vi "Triggers-Stop.vi"(7 "Logging queue element":T1={"Imaging Protocol"=enum."Live Imaging", "Number of Trials"=0, "Frame Size"=512, "# Averaged frames"=0, "Dwell time (us)"=0.0, "Index of Z-plane"=0, "Timelapse?"=FALSE, "Logging process is active"=FALSE, "Speed logging enabled"=FALSE, "tdms file ref"=refnum, "path"=path "", "Trial Number"=0, "Expected # points acquired"=FALSE, "Manually stopped"=FALSE, "Ch0 data"=[], "Ch1 data"=[], "Last trial"=FALSE, "Points acquired"={"Ch0 last trial"=0, "Ch1 last trial"=0, "All trials"=0}} {"Frame Size" items=["100X100"=100, "128X128"=128, "200X200"=200, "256X256"=256, "512X512"=512, "1024x1024"=1024, "2048x2048"=2048]; "Dwell time (us)" format="%#.6g"}, 8 "error in (no error)":errorcluster, 11 "FPGA Ref":T5) -> (0 "error out":errorcluster)   [LabVIEW 2013]
uses:
  RIG-SPECIFIC FILES/FPGA Refs/FPGA Ref.ctl
  Typedefs/Logging queue element.ctl
  Typedefs/Imaging Protocols enum.ctl
  Typedefs/Frame Size.ctl
  Typedefs/Acquired points count.ctl
  Typedefs/Read Write Enum.ctl
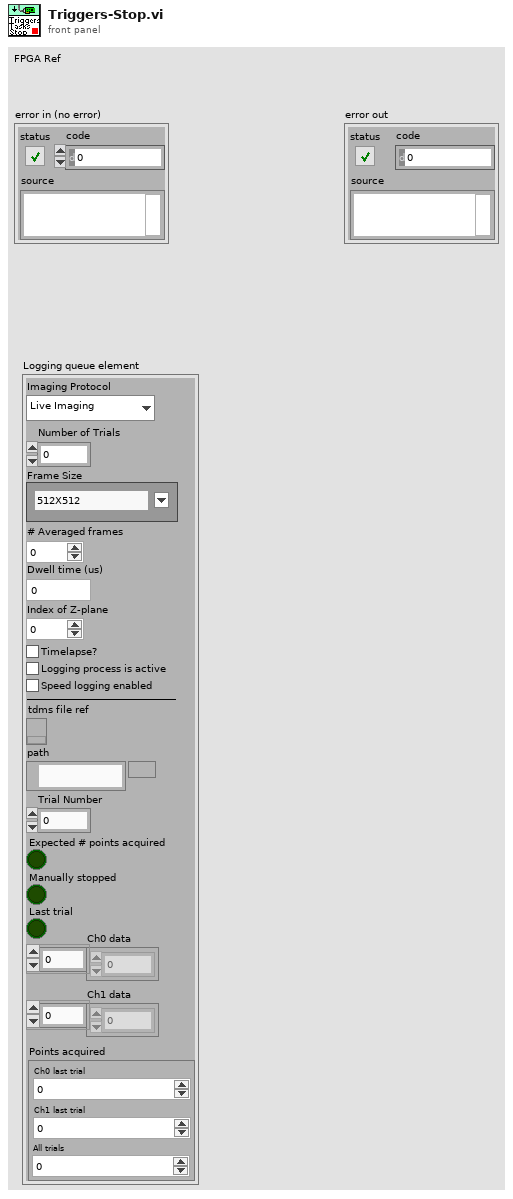
[diagram p1: front panel]
types:
  T1 = typedef "Logging queue element.ctl" = cluster{"Imaging Protocol":T2, "Number of Trials":u16, "Frame Size":T3, "# Averaged frames":u16, "Dwell time (us)":dbl, "Index of Z-plane":i32, "Timelapse?":bool, "Logging process is active":bool, "Speed logging enabled":bool, "tdms file ref":refnum<k34>, "path":path, "Trial Number":i32, "Expected # points acquired":bool, "Manually stopped":bool, "Ch0 data":u32[], "Ch1 data":u32[], "Last trial":bool, "Points acquired":T4}
  T2 = typedef "Imaging Protocols enum.ctl" = enum16{"AOL Z-Stack", "Motor Z Stack", "Functional Acquisition", "Single Plane Acquisition", "Volume Acquisition", "Live Imaging", "Live Plane Imaging", "Live Volume Imaging"}
  T3 = typedef "Frame Size.ctl" = u16
  T4 = typedef "Acquired points count.ctl" = cluster{"Ch0 last trial":u64, "Ch1 last trial":u64, "All trials":u64}
  T5 = typedef "FPGA Ref.ctl" = refnum<k20>
  T6 = typedef "Read Write Enum.ctl" = enum16{"Read", "Write"}
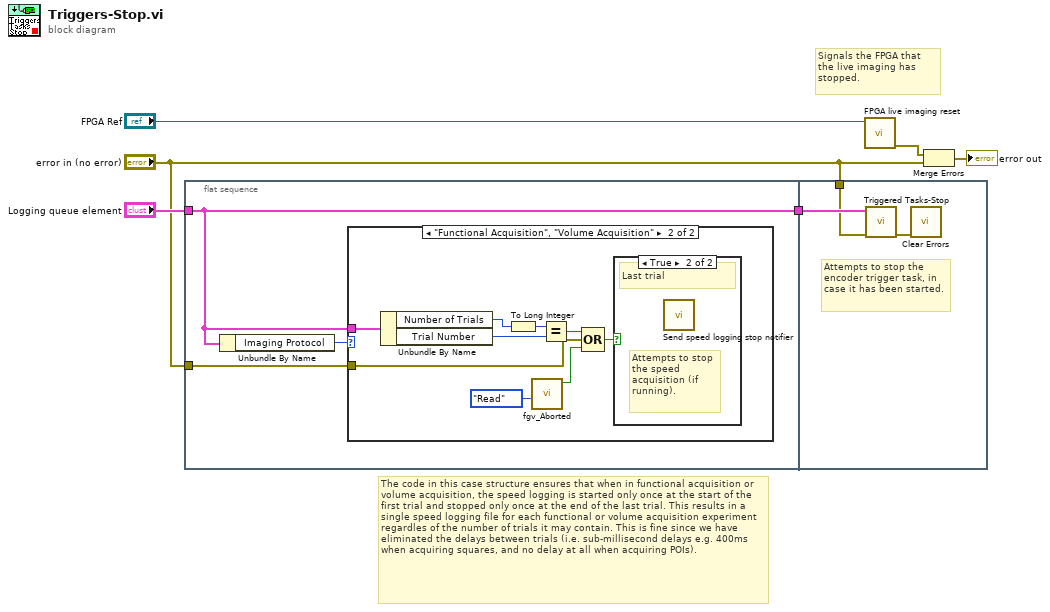
[diagram p0: block diagram]
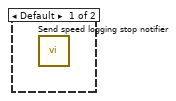
[diagram p2: hidden frame]
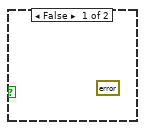
[diagram p3: hidden frame]
diagram:
  # "The code in this case structure ensures that when in functional acquisition or volume acquisition, the speed logging is started only once at the start of the first trial and stopped only once at the end of the last trial. This results in a single speed logging file for each functional or volume acquisition experiment regardles of the number of trials it may contain. This is fine since we have eliminated the delays between trials (i.e. sub-millisecond delays e.g. 400ms when acquiring squares, and no delay at all when acquiring POIs)."
  # "Signals the FPGA that the live imaging has stopped."
  n1 = flat-sequence {
    tunnel: "Logging queue element" -> [w7]
    tunnel: "error in (no error)" -> [w8]
    tunnel: [w7] -> w2
    tunnel: w2 -> [w20]
    tunnel: "error in (no error)" -> [w19]
    frame #0 {
      n2 = Unbundle By Name(w7) -> ("Imaging Protocol"=w9:T2)
      n3 = case shown="\"Functional Acquisition\", \"Volume Acquisition\"" w9 {
        tunnel: w7 -> [_ w15]
        tunnel: w8 -> [_ w11]
        frame Default {
          n4 = call "Send speed logging stop notifier.vi"() -> ()  [unwired: 11 in, 1 out]
        }
        frame "Functional Acquisition", "Volume Acquisition" {
          n5 = Unbundle By Name(w15) -> ("Number of Trials"=w17:u16, "Trial Number"=w18:i32)
          n6 = To Long Integer(number=w17) -> (32bit integer=w16:i32)
          n7 = call "fgv_Aborted.vi"("Function"=Read_Write_Enum."Read") -> ("Funct Acq Aborted?"=w10:bool)  [unwired: 9 in, 1 out]
          n8 = Equal?(x=w16, y=w18) -> (x = y?=w13:bool)
          n9 = Compound Arithmetic op=OR(w13, w11, w10) -> (w12:bool)
          n10 = case shown="True" w12 {
            frame False {
              (unwired) errorcluster {"status"=FALSE, "code"=0, "source"=""} ("error out (No error)")
            }
            frame True {
              # "Attempts to stop the speed acquisition (if running)."
              # "Last trial"
              n11 = call "Send speed logging stop notifier.vi"() -> ()  [unwired: 11 in, 1 out]
            }
          }
        }
      }
    }
    frame #1 {
      # "Attempts to stop the\nencoder trigger task, in \ncase it has been started."
      n12 = call "Triggered Tasks-Stop.vi"("error in (no error)"=w19, "Logging queue element"=w20) -> ("error out"=w21:errorcluster)  [unwired: 9 in]
      n13 = call <vilib>:"Clear Errors.vi"("error in (no error)"=w21) -> ()  [unwired: 6 in, 1 out]
    }
  }
  n14 = call "FPGA live imaging reset.vi"("FPGA VI Ref"="FPGA Ref") -> ("error out"=w5:errorcluster)  [unwired: 10 in]
  n15 = Merge Errors(w5, "error in (no error)") -> (→"error out":errorcluster)
